vi "RPC Method Query.vi"(8 "error in (no error)":errorcluster, 11 "OOP Server in":refnum<class "OCVTest.lvclass">) -> (0 "error out":errorcluster, 3 "OOP Server out":refnum<class "OCVTest.lvclass">)   [LabVIEW 2019, in "OCVTest.lvlib" / "OCVTest.lvclass"]
uses:
  OCVTest.lvclass
  OCVTest.lvclass/OCVTest.ctl
  RPC Messages/measurementservice_QueryResponse/measurementservice_QueryResponse_Data.ctl
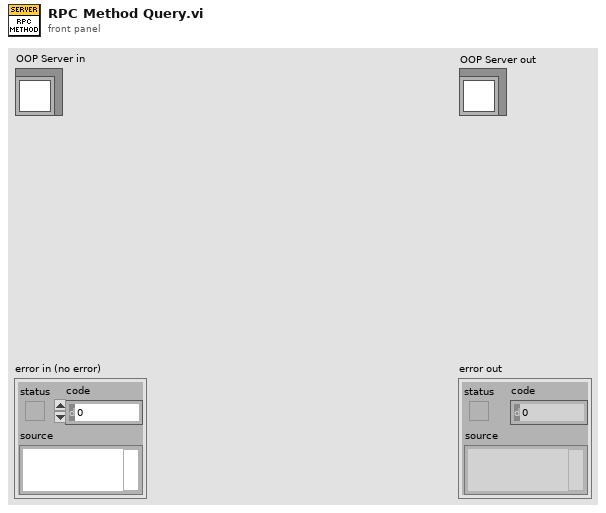
[diagram p1: front panel]
types:
  T1 = typedef "OCVTest.lvlib/OCVTest.lvclass/measurementservice_QueryResponse_Data.ctl" = cluster{"message":string, "status":i32}
  T2 = typedef "OCVTest.lvlib/OCVTest.lvclass/Server Internal UEs.ctl" = cluster{"Invoke Internal UE":refnum<user-event>, "Query Internal UE":refnum<user-event>, "PerformOCVMeasurement Internal UE":refnum<user-event>, "PerformACIRMeasurement Internal UE":refnum<user-event>, "StreamOCVMeasurement Internal UE":refnum<user-event>, "Register Internal UE":refnum<user-event>}
  T3 = typedef "OCVTest.lvlib/OCVTest.lvclass/Server gRPC UEs.ctl" = cluster{"Invoke gRPC UE":refnum<user-event>, "Query gRPC UE":refnum<user-event>, "PerformOCVMeasurement gRPC UE":refnum<user-event>, "PerformACIRMeasurement gRPC UE":refnum<user-event>, "StreamOCVMeasurement gRPC UE":refnum<user-event>, "Register gRPC UE":refnum<user-event>}
  T4 = typedef "OCVTest.lvlib/gprc-lvsupport.lvlib/grpcId.ctl" = u64
  T5 = typedef "OCVTest.lvlib/OCVTest.lvclass/measurementservice_QueryRequest_Data.ctl" = cluster{"query":string}
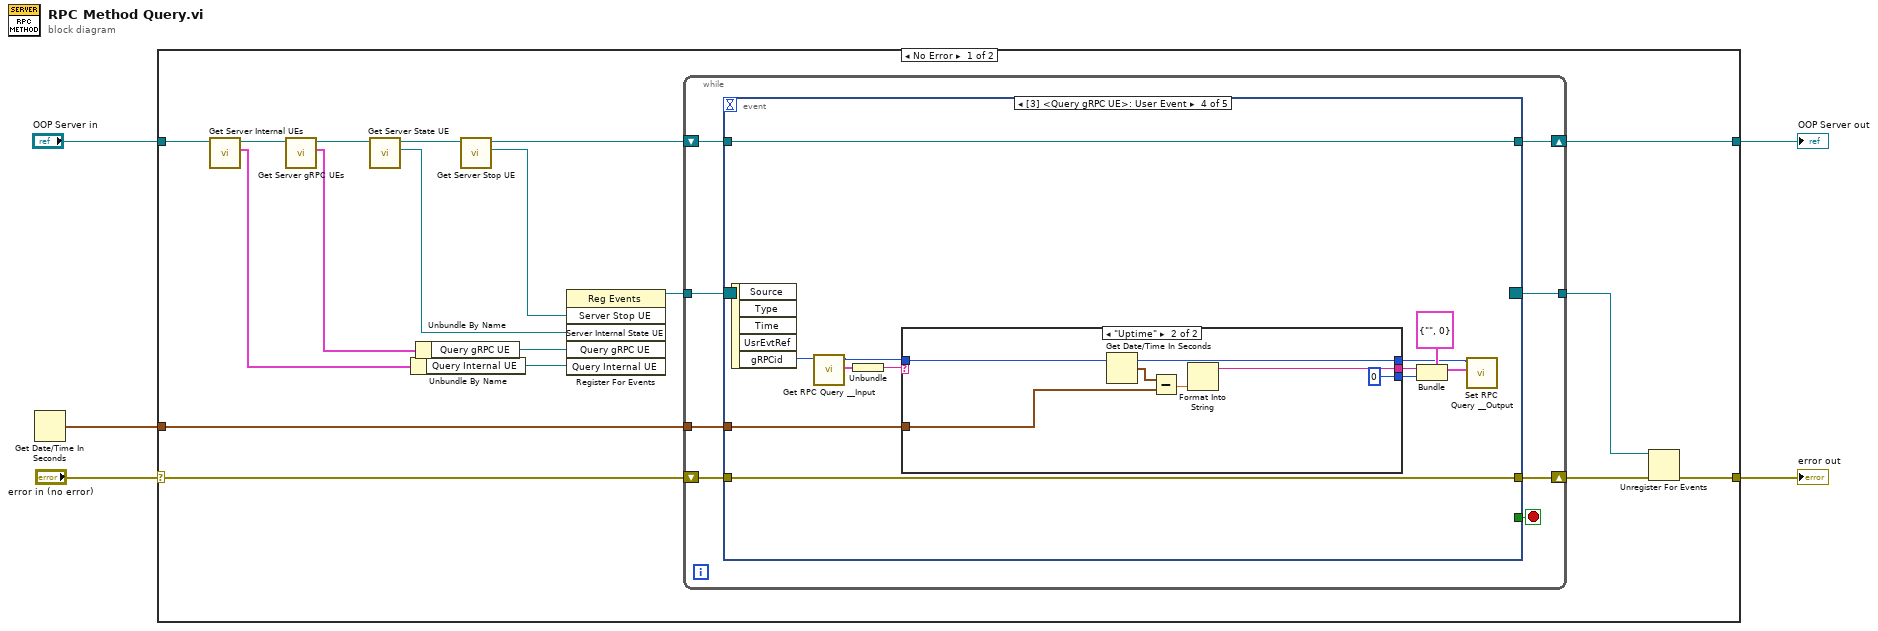
[diagram p0: block diagram]
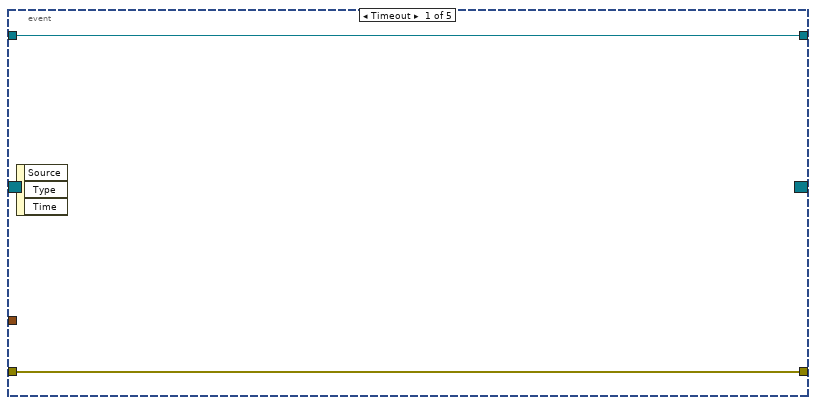
[diagram p2: hidden frame]
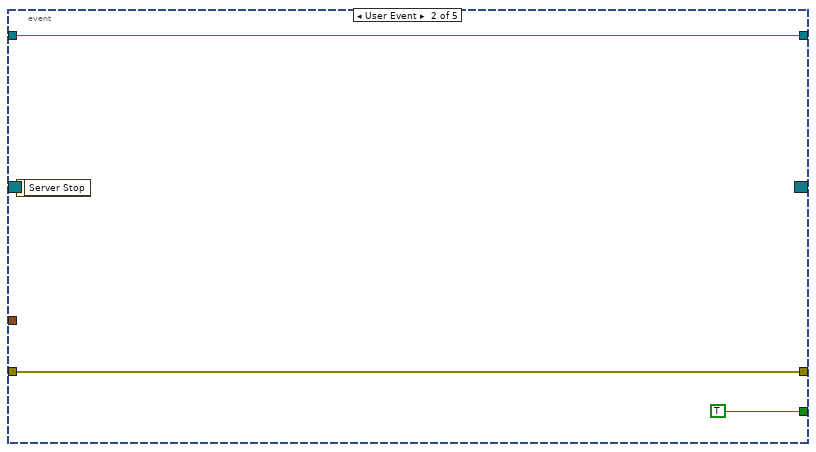
[diagram p3: hidden frame]
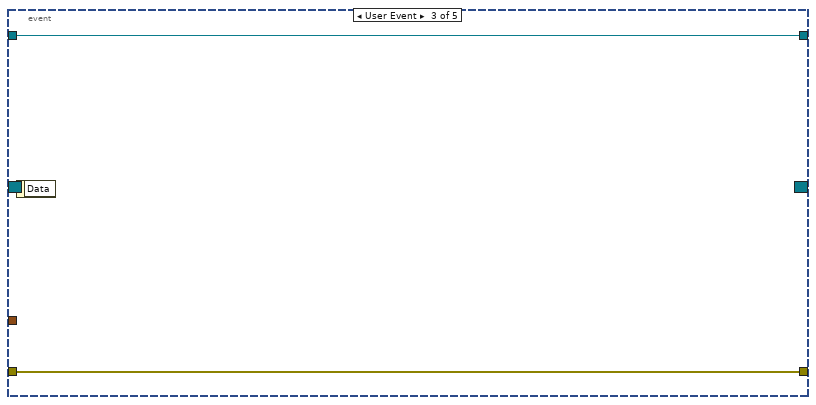
[diagram p4: hidden frame]
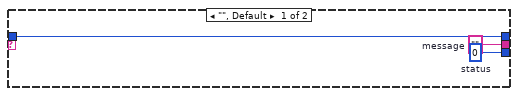
[diagram p5: hidden frame]
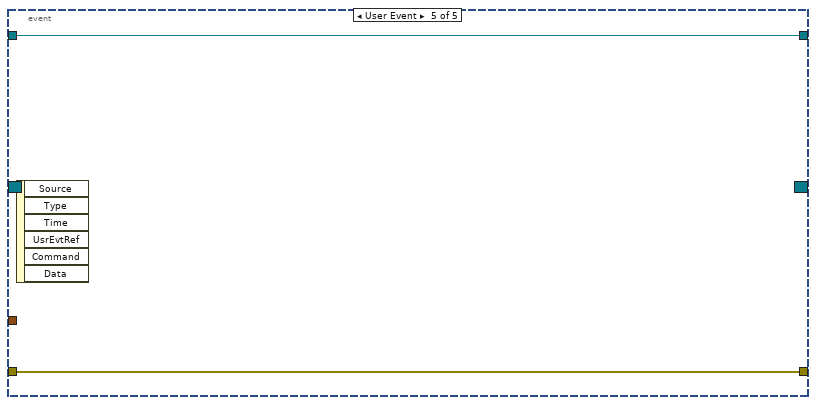
[diagram p6: hidden frame]
diagram:
  n1 = Get Date/Time In Seconds() -> (seconds since 1Jan1904=w1:timestamp)
  n2 = case shown="No Error" "error in (no error)" {
    selector: "error in (no error)" -> [w19 w63]
    tunnel: [w17 w63] -> w4
    tunnel: "OOP Server in" -> [w21 w62]
    tunnel: [w7 w62] -> w2
    tunnel: w1 -> [w6 _]
    frame No Error {
      n3 = call "Get Server Internal UEs.vi"("OOP Server in"=w21) -> ("Server Internal UEs"=w13:T2, "OOP Server out"=w20:refnum<class "OCVTest.lvclass">)  [unwired: 9 in]
      n4 = call "Get Server gRPC UEs.vi"("OOP Server in"=w20) -> ("Server gRPC UEs"=w15:T3, "OOP Server out"=w10:refnum<class "OCVTest.lvclass">)  [unwired: 9 in]
      n5 = call "Get Server State UE.vi"("Template Server in"=w10) -> ("Server Internal State UE"=w8:refnum<user-event>, "Template Server out"=w9:refnum<class "OCVTest.lvclass">)  [unwired: 9 in]
      n6 = Unbundle By Name ("Unbundle Internal UE")(w13) -> ("Query Internal UE"=w12:refnum<user-event>)
      n7 = Unbundle By Name ("Unbundle gRPC UE")(w15) -> ("Query gRPC UE"=w14:refnum<user-event>)
      n8 = call "Get Server Stop UE.vi"("OOP Server in"=w9) -> ("Server Stop UE"=w23:refnum<user-event>, "OOP Server out"=w11:refnum<class "OCVTest.lvclass">)  [unwired: 9 in]
      n9 = register-events(w23, w8, w14, w12) -> (reference out=w22:refnum<event-registration>)  [unwired: 2 in, 1 out]
      n10 = while {
        tunnel: w22 -> [w31]
        tunnel: [w27] -> w16
        shift-right: [w28] -> w18
        shift-left: w19 -> [w29]
        shift-right: [w25] -> w7
        shift-left: w11 -> [w26]
        tunnel: w6 -> [w24]
        stop <- w30 stop-if-true
        n11 = event "RPC Method Event Structure" shown="[3] <Query gRPC UE>: User Event" {
          selector: w31 -> [_ _ _ _ _]
          dyn-events: [_ _ _ _ _] -> w27
          timeout: _ -> [_ _ _ _ _]
          tunnel: [_ TRUE _ _ _] -> w30
          tunnel: w29 -> [w33 w35 w38 w50 w61]
          tunnel: [w33 w35 w38 w50 w61] -> w28
          tunnel: w26 -> [w32 w34 w37 w49 w60]
          tunnel: [w32 w34 w37 w49 w60] -> w25
          tunnel: w24 -> [_ _ _ w44 _]
          event Timeout {
            n12 = event-data() -> ()  [unwired: 1 in, 3 out]
          }
          event User Event {
            n13 = event-data() -> ()  [unwired: 1 in, 1 out]
          }
          event User Event {
            n14 = event-data() -> ()  [unwired: 1 in, 1 out]
          }
          event User Event {
            n15 = event-data() -> ("gRPCid"=w43:T4)  [unwired: 1 in, 4 out]
            n16 = call "Get RPC Query __Input.vi"("gRPCid in"=w43) -> ("Message Data"=w41:T5, "gRPCid out"=w42:T4)  [unwired: 8 in, 1 out]
            n17 = Unbundle(w41) -> ("query"=w48:string)
            n18 = case shown="\"Uptime\"" w48 {
              tunnel: w42 -> [w53 w56]
              tunnel: [w53 w56] -> w40
              tunnel: [w52 w57] -> w46
              tunnel: [w51 0 ("status")] -> w45
              tunnel: w44 -> [_ w54]
              frame "", Default {
                w51 = 0  # status
                w52 = ""  # message
              }
              frame "Uptime" {
                n19 = Get Date/Time In Seconds() -> (seconds since 1Jan1904=w59:timestamp)
                n20 = Subtract(x=w59, y=w54) -> (x-y=w58:dbl)
                n21 = Format Into String(w58) -> (resulting string=w57:string)  [unwired: 3 in, 1 out]
              }
            }
            n22 = Bundle(cluster=T1 {"message"="", "status"=0} ("Message Data"), "message"=w46, "status"=w45) -> (w39:T1)
            n23 = call "Set RPC Query __Output.vi"("Message Data"=w39, "gRPCid in"=w40) -> ()  [unwired: 9 in, 1 out]
          }
          event User Event {
            n24 = event-data() -> ()  [unwired: 1 in, 6 out]
          }
        }
      }
      n25 = Unregister For Events(event registration refnum=w16, error in=w18) -> (error out=w17:errorcluster)
    }
    frame Error {
    }
  }
  "error out" <- w4
  "OOP Server out" <- w2
